vi "GA Cmp Buf Data.vi"(0 "nCmpEncodeNum":i16, 1 "nPluseType":i16, 2 "nStartLevel":i16, 3 "nTime":i16, 4 "pBuf1":i32, 5 "nBufLen1":i16, 6 "pBuf2":i32, 7 "error in (no error)":errorcluster caption="错误输入（无错误）", 8 "nBufLen2":i16, 9 "nAbsPosFlag":i16, 10 "nTimerFlag":i16) -> (20 "function return":i32, 24 "pBuf1 out":i32, 26 "pBuf2 out":i32, 27 "error out":errorcluster caption="错误输出")   [LabVIEW 2015, in "GAS.lvlib"]
doc: "extern \"C\" __declspec(dllimport) int GA_CmpBufData(short nCmpEncodeNum, short nPluseType, short nStartLevel, short nTime, long *pBuf1, short nBufLen1, long *pBuf2, short nBufLen2,short nAbsPosFlag=0,short nTimerFlag=0);"
uses:
  <userlib>/BP_GAS/GAS.lvlib
  <userlib>/BP_GAS/GAS.dll
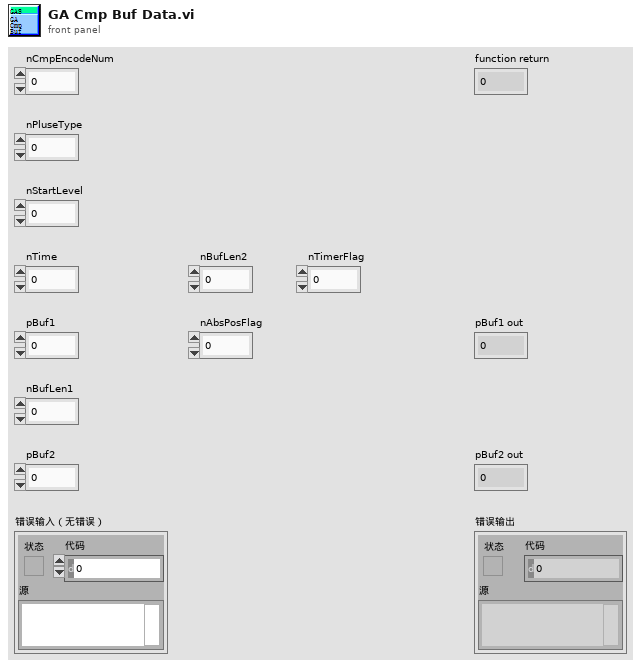
[diagram p1: front panel]
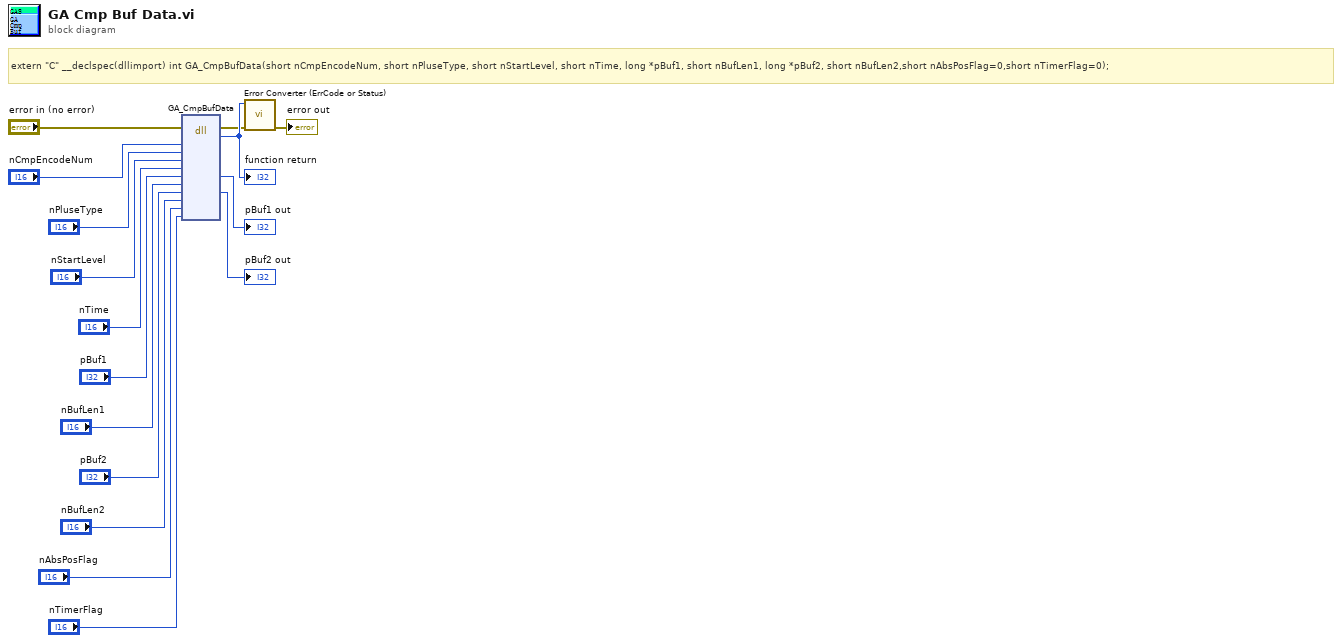
[diagram p0: block diagram]
diagram:
  # "extern \"C\" __declspec(dllimport) int GA_CmpBufData(short nCmpEncodeNum, short nPluseType, short nStartLevel, short nTime, long *pBuf1, short nBufLen1, long *pBuf2, short nBufLen2,short nAbsPosFlag=0,short nTimerFlag=0);"
  n1 = dll-call lib="E:/Program Files (x86)/National Instruments/LabVIEW 2015/user.lib/BP_GAS/GAS.*" fn="GA_CmpBufData"(error in="error in (no error)", "nCmpEncodeNum"="nCmpEncodeNum", "nPluseType"="nPluseType", "nStartLevel"="nStartLevel", "nTime"="nTime", "pBuf1"="pBuf1", "nBufLen1"="nBufLen1", "pBuf2"="pBuf2", "nBufLen2"="nBufLen2", "nAbsPosFlag"="nAbsPosFlag", "nTimerFlag"="nTimerFlag") -> (error out=w2:errorcluster, w16:i32, "pBuf1"=→"pBuf1 out":i32, "pBuf2"=→"pBuf2 out":i32)  [unwired: 10 in, 1 out]
  "function return" <- w16
  n2 = call "Error Converter (ErrCode or Status).vi"("error in (no error)"=w2, "error code"=w16) -> ("error out"=→"error out":errorcluster)  [unwired: 9 in]
